vi "TR_GEN_Location-based_density_map.vi"(0 "Overlays cluster in":T2, 5 "XY data":T3, 7 "Post-processing parameters":variant, 9 "Image transformation parameters":T1={"Input array is image? (F)"=FALSE, "Log2-transform? (T)"=TRUE, "Normalize to 8 bit? (T)"=TRUE, "Output as Image? (T)"=TRUE}, 11 "error in (no error)":errorcluster) -> (4 "Overlays cluster out":T2, 15 "error out":errorcluster)   [LabVIEW 2018, in "Tracks Repair.lvlib"]
uses:
  Tracks Repair.lvlib
  SubVi's/Controls/CTL_Full_Track_Array.ctl
  SubVi's/Controls/CTL_Overlays_cluster.ctl
  SubVi's/Controls/CTL_2D_bins_parameters.ctl
  SubVi's/Controls/CTL_Post-processing_params.ctl
  SubVi's/Controls/CTL_Filter_selector.ctl
  SubVi's/Controls/CTL_Mouse_Draw_Params.ctl
  <vilib>/vision/Image Controls.llb/IMAQ Image.ctl
  SubVi's/Controls/CTL_Calibration_parameters.ctl
  SubVi's/Controls/CTL_Dispenser_calibration_info.ctl
  SubVi's/Controls/CTL_Pixel_to_Zone_array.ctl
  SubVi's/Controls/CTL_Color_ramp.ctl
  SubVi's/Calc and data manipulation/GET_2D_Data_Binning_(location).vi
  Tracker.lvlib
  Common_Resources.lvlib
panel:
  out "Interp. size":i32[](array[numeric])
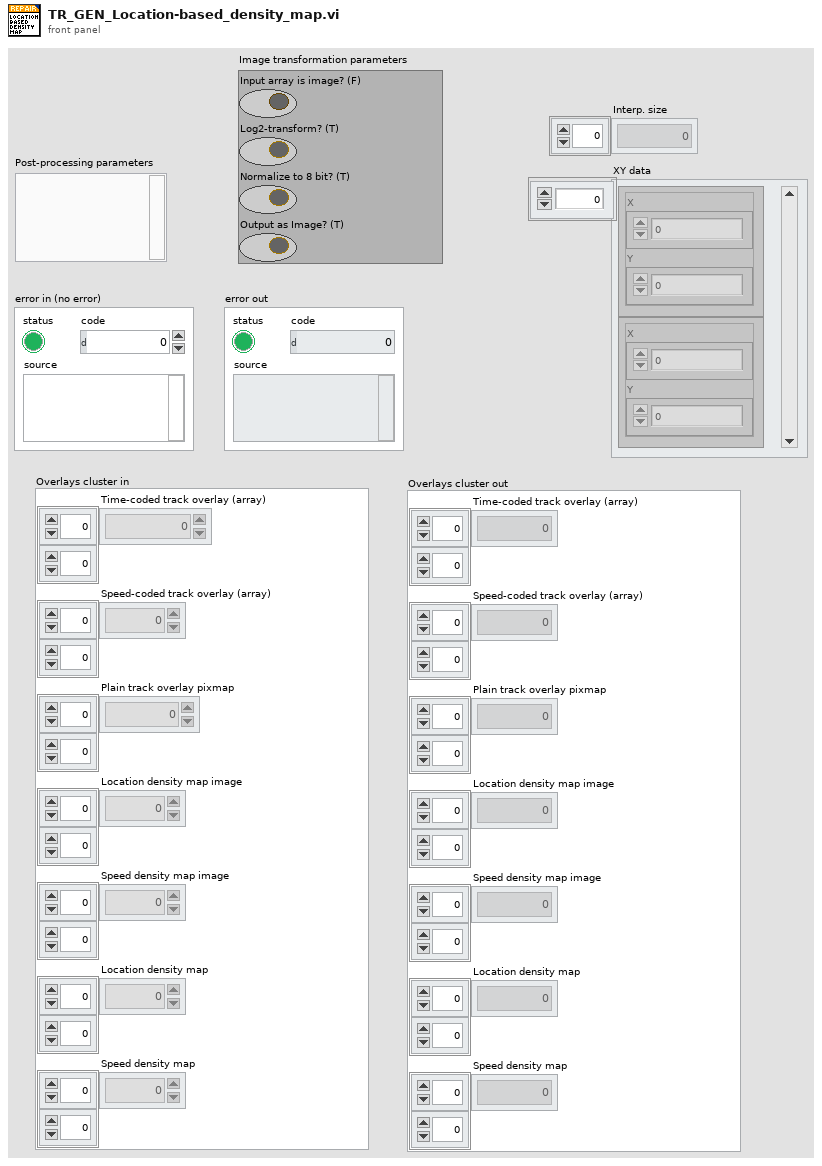
[diagram p1: front panel]
types:
  T1 = cluster{"Input array is image? (F)":bool, "Log2-transform? (T)":bool, "Normalize to 8 bit? (T)":bool, "Output as Image? (T)":bool}
  T2 = typedef "Common_Resources.lvlib/CTL_Overlays_cluster.ctl" = cluster{"Time-coded track overlay (array)":u32[][], "Speed-coded track overlay (array)":u32[][], "Plain track overlay pixmap":u32[][], "Location density map image":u32[][], "Speed density map image":u32[][], "Location density map":dbl[][], "Speed density map":dbl[][]}
  T3 = typedef "Common_Resources.lvlib/CTL_Full_Track_Array.ctl" = cluster{"X":dbl, "Y":dbl}[]
  T4 = typedef "Common_Resources.lvlib/CTL_Post-processing_params.ctl" = cluster{"Defragment TDMS? (F)":bool, "Start time (SW)":timestamp, "Start time (HW)":u32, "Data filtering":T5, "Mouse drawing parameters":T6, "Size of the image (480x480)":cluster{"X size":dbl, "Y size":dbl}, "Image ref. in":T7, "Calibration parameters":T8, "Pixel to zone":T10}
  T5 = typedef "Common_Resources.lvlib/CTL_Filter_selector.ctl" = cluster{"Filter type":enum16{"None", "Savitzky-Golay"}, "Length":i32, "Order":i32}
  T6 = typedef "Common_Resources.lvlib/CTL_Mouse_Draw_Params.ctl" = cluster{"Trace length, samples":u16, "Rainbow track":bool, "Rainbow track is speed":bool, "Bright mouse lineout":bool, "Colors array":u32[], "Pixels per mm":dbl}
  T7 = typedef "IMAQ Image.ctl" = refnum<image>
  T8 = typedef "Common_Resources.lvlib/CTL_Calibration_parameters.ctl" = cluster{"Timing calibration sw/hw":dbl, "True FPS":dbl, "True frame time, s":dbl, "Disp. calibration info":T9}
  T9 = typedef "Common_Resources.lvlib/CTL_Dispenser_calibration_info.ctl" = cluster{"Channel":u8, "Speed, µl per ms":dbl}[]
  T10 = typedef "Common_Resources.lvlib/CTL_Pixel_to_Zone_array.ctl" = i8[][]
  T11 = typedef "Common_Resources.lvlib/CTL_2D_bins_parameters.ctl" = cluster{"Xmax":dbl, "Xmin":dbl, "Ymax":dbl, "Ymin":dbl, "# bins per axis":i32}
  T12 = typedef "Common_Resources.lvlib/CTL_Color_ramp.ctl" = u32[]
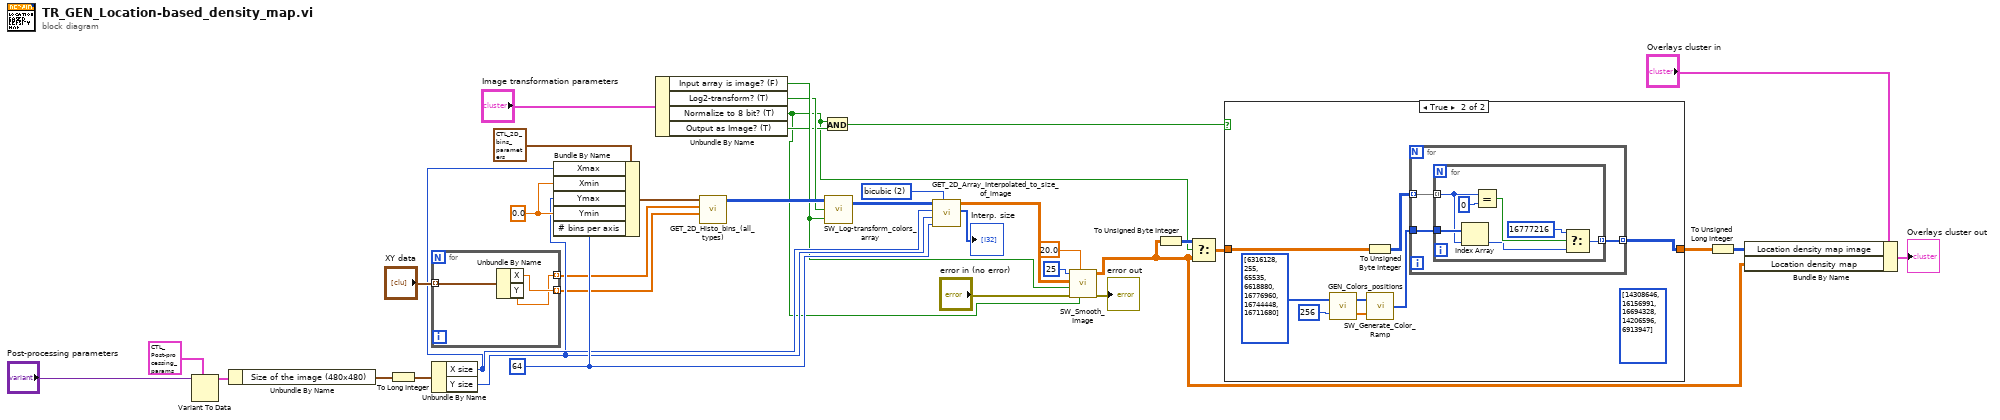
[diagram p0: block diagram]
diagram:
  w28 = 2 items=["nearest", "bilinear", "bicubic", "bicubic spline"] ("Method")
  w27 = 64 ("# bins per axis")
  w30 = 0.0 ("Xmin")
  n1 = Variant To Data(type=T4 {"Defragment TDMS? (F)"=FALSE, "Start time (SW)"=timestamp(0 s since 1904-01-01), "Start time (HW)"=0, "Data filtering"={"Filter type"=enum."Savitzky-Golay", "Length"=41, "Order"=3}, "Mouse drawing parameters"={"Trace length, samples"=0, "Rainbow track"=FALSE, "Rainbow track is speed"=FALSE, "Bright mouse lineout"=FALSE, "Colors array"=[], "Pixels per mm"=0.0}, "Size of the image (480x480)"={"X size"=480.0, "Y size"=480.0}, "Image ref. in"=refnum, "Calibration parameters"={"Timing calibration sw/hw"=1.0, "True FPS"=80.0, "True frame time, s"=0.0125, "Disp. calibration info"=[]}, "Pixel to zone"=[]} ("Processing parameters"), Variant="Post-processing parameters") -> (data=w13:T4)  [unwired: 1 in, 1 out]
  n2 = Unbundle By Name(w13) -> ("Size of the image (480x480)"=w12:cluster{"X size":dbl, "Y size":dbl})
  n3 = To Long Integer(number=w12) -> (32bit integer=w11:cluster{"X size":i32, "Y size":i32})
  n4 = for {
    tunnel: "XY data" -> [w39] mode=indexing
    tunnel: [w38] -> w19 mode=indexing
    tunnel: [w37] -> w18 mode=indexing
    n5 = Unbundle By Name(w39) -> ("X"=w38:dbl, "Y"=w37:dbl)
  }
  n6 = Unbundle By Name(w11) -> ("X size"=w21:i32, "Y size"=w20:i32)
  n7 = Bundle By Name(cluster=T11 {"Xmax"=110.0, "Xmin"=-110.0, "Ymax"=110.0, "Ymin"=-110.0, "# bins per axis"=64} ("Bins parameters"), "Xmax"=w21, "Xmin"=w30, "Ymax"=w20, "Ymin"=w30, "# bins per axis"=w27) -> (w31:T11)
  n8 = Unbundle By Name("Image transformation parameters") -> ("Input array is image? (F)"=w4:bool, "Log2-transform? (T)"=w3:bool, "Normalize to 8 bit? (T)"=w1:bool, "Output as Image? (T)"=w2:bool)
  n9 = call-poly "GET_2D_Histo_bins_(all_types).vi"("X"=w19, "Y"=w18, "Bins parameters"=w31) -> ("Binned array"=w17:u32[][])  [unwired: 3 in]
  n10 = And(x=w1, y=w2) -> (x .and. y?=w23:bool)
  n11 = call "SW_Log-transform_colors_array.vi"("Image? (T)"=w4, "Log-transform? (F)"=w3, "Array or 24-bit pixmap in"=w17) -> ("Array or 24-bit pixmap out"=w16:u32[][])  [unwired: 1 in]
  n12 = call "GET_2D_Array_Interpolated_to_size_of_image.vi"("Method"=w28, "# bins per axis"=w27, "Y image size"=w20, "X image size"=w21, "Array or pixmap in"=w16) -> ("Interp. size"=→"Interp. size":i32[], "Array or pixmap out"=w22:dbl[][])  [unwired: 5 in]
  n13 = call "SW_Smooth_Image.vi"("Normalize to 8-bit range? (T)"=w1, "Sigma"=20.0, "Error In"="error in (no error)", "Image? (T)"=w4, "Array or pixmap in"=w22, "Kernel size"=u32 25) -> ("Error Out"=→"error out":errorcluster, "Array or pixmap out"=w6:dbl[][])  [unwired: 4 in]
  n14 = To Unsigned Byte Integer(number=w6) -> (unsigned 8bit integer=w25:u8[][])
  n15 = Select(t=w25, s=w1, f=w6) -> (s? t:f=w24:dbl[][])
  n16 = case shown="True" w23 {
    tunnel: [w40 w42] -> w9
    tunnel: w24 -> [w40 w48]
    frame False {
    }
    frame True {
      (unwired) u32[] [14308646, 16156991, 16694328, 14206596, 6913947] ("Initial colors ramp array")
      n17 = call "GEN_Colors_positions.vi"("Highest color position"=u32 256, "Initial colors ramp array in"=T12 [6316128, 255, 65535, 6618880, 16776960, 16744448, 16711680] ("Initial colors ramp array")) -> ("Colors positions"=w47:dbl[], "Initial colors ramp array out"=w46:T12)
      n18 = To Unsigned Byte Integer(number=w48) -> (unsigned 8bit integer=w45:u8[][])
      n19 = call "SW_Generate_Color_Ramp.vi"("Colors rel. pos."=w47, "Colors array"=w46) -> ("Colors array"=w43:u32[])
      n20 = for {
        tunnel: w45 -> [w51] mode=indexing
        tunnel: [w50] -> w42 mode=indexing
        tunnel: w43 -> [w49]
        n21 = for {
          tunnel: w51 -> [w55] mode=indexing
          tunnel: [w52] -> w50 mode=indexing
          tunnel: w49 -> [w58]
          n22 = Index Array(array=w58, index=w55) -> (element=w53:u32)
          n23 = Equal?(x=w55, y=0) -> (x = y?=w56:bool)
          n24 = Select(t=16777216, s=w56, f=w53) -> (s? t:f=w52:u32)
        }
      }
    }
  }
  n25 = To Unsigned Long Integer(number=w9) -> (unsigned 32bit integer=w8:u32[][])
  n26 = Bundle By Name(cluster="Overlays cluster in", "Location density map image"=w8, "Location density map"=w6) -> (→"Overlays cluster out":T2)
